vi "Determine photogate shutter logic.vi"(2 "Acquisition mode":enum32{"Continuous", "Time-lapse"}(ring), 3 "Shutter open/close  time (ms)":sgl, 4 "Exposure(ms)":sgl, 5 "Kinetic cycle time (ms)":sgl) -> (1 "Photogate shutter\nsync possible":bool)   [LabVIEW 2011]
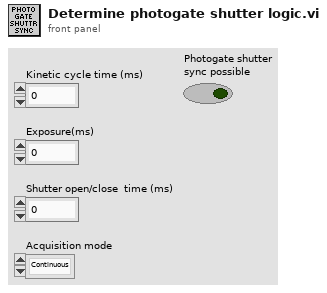
[diagram p1: front panel]
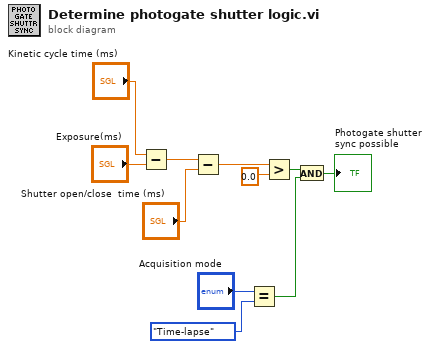
[diagram p0: block diagram]
diagram:
  n1 = Subtract(x="Kinetic cycle time (ms)", y="Exposure(ms)") -> (x-y=w5:sgl)
  n2 = Subtract(x=w5, y="Shutter open/close  time (ms)") -> (x-y=w7:sgl)
  n3 = Equal?(x="Acquisition mode", y=enum32{"Continuous", "Time-lapse"}."Time-lapse" ("Acquisition mode")) -> (x = y?=w10:bool)
  n4 = Greater?(x=w7, y=sgl 0.0) -> (0:w9:bool)
  n5 = And(x=w9, y=w10) -> (x .and. y?=→"Photogate shutter\nsync possible":bool)
